vi "OpenCVFaceDetection_ClassCast.vi"(11 "OpenCVFaceDetectionIn":refnum<class>) -> (3 "OpenCVFaceDetectionOut":refnum<class "OpenCVFaceDetection.lvclass">)   [LabVIEW 2021, in "OpenCVFaceDetection.lvclass"]
uses:
  OpenCVFaceDetection.lvclass
  OpenCVFaceDetection.lvclass/OpenCVFaceDetection.ctl
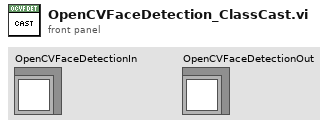
[diagram p1: front panel]
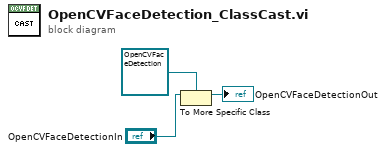
[diagram p0: block diagram]
diagram:
  n1 = To More Specific Class(target class=refnum<class "OpenCVFaceDetection.lvclass"> refnum ("reference in"), reference="OpenCVFaceDetectionIn") -> (specific class reference=→"OpenCVFaceDetectionOut":refnum<class "OpenCVFaceDetection.lvclass">)  [unwired: 1 in, 1 out]
